vi "Set Light.vi"   [LabVIEW 2017, in "NI_3D Picture Control.lvlib"]
doc: "Creates and positions a light source in 3D space relative to a 3D object."
uses:
  <vilib>/picture/3D Picture Control/NI_3D Picture Control.lvlib
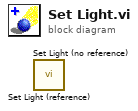
[diagram p0: block diagram]
diagram:
  n1 = call <vilib>:"Set Light (reference).vi"() -> ()  [unwired: 9 in, 3 out]
  n2 = call <vilib>:"Set Light (no reference).vi"() -> ()  [unwired: 10 in, 2 out]
